vi "String Parsing Implementation.vi"(8 "error in (no error)":errorcluster, 11 "class path":path) -> (0 "error out":errorcluster, 3 "Array":path[](array[path]))   [LabVIEW 2020, in "Test Method Finding Test.lvclass"]
uses:
  Test Method Finding Test.lvclass
  Test Method Finding Test.lvclass/Test Method Finding Test.ctl
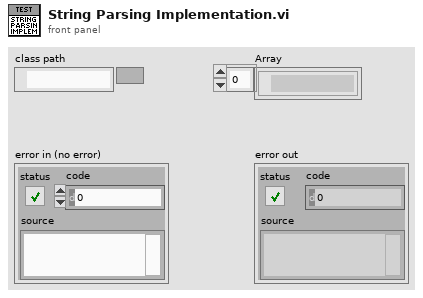
[diagram p1: front panel]
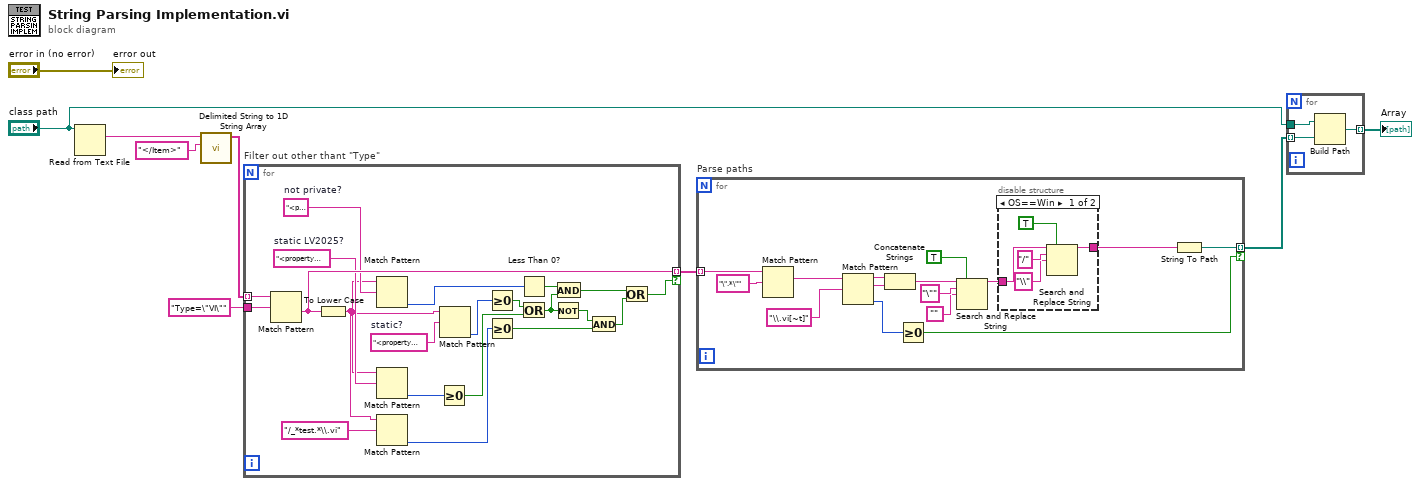
[diagram p0: block diagram]
diagram:
  n1 = Read from Text File(file (use dialog)="class path") -> (text=w8:string)  [unwired: 3 in, 3 out]
  n2 = call <vilib>:"Delimited String to 1D String Array.vi"("delimiter"="</Item>" ("regular expression"), "delimited string"=w8) -> ("string array"=w1:string[])  [unwired: 9 in]
  n3 = for "Filter out other thant \"Type\"" {
    tunnel: w1 -> [w30] mode=indexing
    tunnel: [w25] -> w3 mode=indexing if=w10
    tunnel: "Type=\"VI\"" ("regular expression") -> [w29]
    w14 = "<property name=\"ni.classitem.invokeusage\" type=\"uint\">0"  # static LV2025?
    w24 = "<property name=\"ni.classitem.methodscope\" type=\"uint\">2"  # not private?
    w28 = "<property name=\"ni.classitem.isstaticmethod\" type=\"bool\">true"  # static?
    n4 = Match Pattern(string=w30, regular expression=w29) -> (after substring=w25:string)  [unwired: 1 in, 3 out]
    n5 = To Lower Case(string=w25) -> (all lower case string=w11:string)
    n6 = Match Pattern(string=w11, regular expression=w24) -> (offset past match=w26:i32)  [unwired: 1 in, 3 out]
    n7 = Match Pattern(string=w11, regular expression=w14) -> (offset past match=w15:i32)  [unwired: 1 in, 3 out]
    n8 = Match Pattern(string=w11, regular expression="/_*test.*\\.vi") -> (offset past match=w21:i32)  [unwired: 1 in, 3 out]
    n9 = Greater Or Equal To 0?(x=w15) -> (x >= 0?=w12:bool)
    n10 = Match Pattern(string=w11, regular expression=w28) -> (offset past match=w27:i32)  [unwired: 1 in, 3 out]
    n11 = Greater Or Equal To 0?(x=w27) -> (x >= 0?=w20:bool)
    n12 = Greater Or Equal To 0?(x=w21) -> (x >= 0?=w18:bool)
    n13 = Less Than 0?(x=w26) -> (x < 0?=w23:bool)
    n14 = Or(x=w20, y=w12) -> (x .or. y?=w13:bool)
    n15 = Not(x=w13) -> (.not. x?=w19:bool)
    n16 = And(x=w23, y=w13) -> (x .and. y?=w17:bool)
    n17 = And(x=w19, y=w18) -> (x .and. y?=w16:bool)
    n18 = Or(x=w17, y=w16) -> (x .or. y?=w10:bool)
  }
  n19 = for "Parse paths" {
    tunnel: w3 -> [w45] mode=indexing
    tunnel: [w40] -> w6 mode=indexing if=w31
    n20 = Match Pattern(string=w45, regular expression="\".*\"") -> (match substring=w35:string)  [unwired: 1 in, 3 out]
    n21 = Match Pattern(string=w35, regular expression="\\.vi[~t]") -> (before substring=w37:string, match substring=w36:string, offset past match=w32:i32)  [unwired: 1 in, 1 out]
    n22 = Concatenate Strings(w37, w36) -> (w34:string)
    n23 = Greater Or Equal To 0?(x=w32) -> (x >= 0?=w31:bool)
    n24 = Search and Replace String(replace all?=TRUE ("replace all? (F)"), input string=w34, search string="\"", replace string="") -> (result string=w39:string)  [unwired: 4 in, 3 out]
    n25 = disable-structure shown="OS==Win" {
      disable-tunnel: [w49 w51] -> w33
      disable-tunnel: w39 -> [w48 w51]
      frame condition #0 (active) {
        n26 = Search and Replace String(replace all?=TRUE ("replace all? (F)"), input string=w48, search string="/", replace string="\\" ("search string")) -> (result string=w49:string)  [unwired: 4 in, 3 out]
      }
      frame condition #1 {
      }
    }
    n27 = String To Path(string=w33) -> (path=w40:path)
  }
  n28 = for {
    tunnel: "class path" -> [w54]
    tunnel: w6 -> [w53] mode=indexing
    tunnel: [w52] -> w5 mode=indexing
    n29 = Build Path(base path=w54, name or relative path=w53) -> (appended path=w52:path)
  }
  "Array" <- w5
  "error out" <- "error in (no error)"
